vi "Master_DAQ_fixGetAverage.vi"(1 "new value":dbl) -> (0 "mean":dbl format="%0.2f")   [LabVIEW 2018]
uses:
  <vilib>/Analysis/baseanly.llb/Mean (DBL).vi
  <vilib>/Analysis/NI_AALBase.lvlib
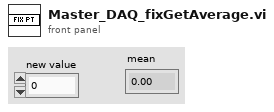
[diagram p1: front panel]
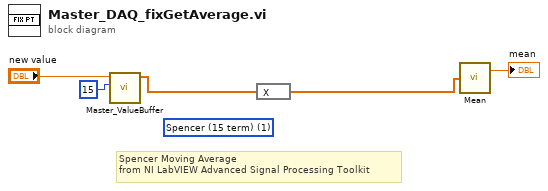
[diagram p0: block diagram]
diagram:
  (unwired) 1 items=["Spencer (15 term)"=1, "Henderson (7 term)"=2, "Henderson (9 term)"=3, "Henderson (13 term)"=4, "Henderson (23 term)"=5] ("method")
  # "Spencer Moving Average \nfrom NI LabVIEW Advanced Signal Processing Toolkit"
  n1 = call "Master_ValueBuffer.vi"("n"=15, "new value"="new value") -> ("Last n values"=w2:dbl[])  [unwired: 9 in]
  n2 = expression code="X"(w2) -> (w1:dbl[])
  n3 = call-poly <vilib>:"Mean.vi"("X"=w1) -> ("mean"=→"mean":dbl)  [unwired: 1 out]
